vi "Host.vi"() -> ()   [LabVIEW 2018]
uses:
  <vilib>/userdefined/High Color/nirio_resource_hc.ctl
  <vilib>/FPGAPlugInAG/PXI-7953R/niLvFpga_Open_PXI-7953R.vi
  <vilib>/rvi/interface/common/dynamic/niFpgaDynamicAddResources.vi
  <vilib>/Utility/error.llb/Error Cluster From Error Code.vi
  <vilib>/rvi/errors/niLvFpgaAdjustHostInterfaceError.vi
  <vilib>/FPGAPlugInAG/Dynamic/niLvFpga_Close_Dynamic.vi
  <vilib>/rvi/interface/nirviOpenFPGA/nirviOpenFPGA.xnode
  FPGA Bitfiles/Memory_FPGATarget_Target_2uGpIeDGXOU.lvbitx
  <vilib>/rvi/interface/nirviReadWriteControl/nirviReadWriteControl.xnode
  <vilib>/rvi/interface/nirviMethod/nirviMethod.xnode
  <vilib>/rvi/interface/nirviCloseFPGA/nirviCloseFPGA.xnode
  <vilib>/FPGAPlugInAG/Dynamic/niLvFpga_ReadFifo_Dynamic.vi
  <vilib>/rvi/errors/niLvFpgaMergeErrorWithErrorCode.vi
  <vilib>/rvi/interface/Simulation/niFpgaSimulationCallBeginRW.vi
  NiFpgaLv.dll
panel:
  out "Data 2":u32[][](array[numeric])
  in  "Requested Number of Elements":u32
  in  "16384":u32
  in  "131":i32
  in  "Чтение всей памяти":bool
  out "Elements Remaining":u32
  out "Number of Elements to Write":u32
  out "Data":u8
  in  "2":u8=2
  in  "4":u8=4
  in  "Address":u32
  in  "Запись в DRAM":bool
  in  "D-0":u32
  in  "Чтение DRAM":bool
  in  "FIFO":bool
  in  "resource name":T1="PXI1Slot5" caption="RIO Device"
  in  "Стоп":bool
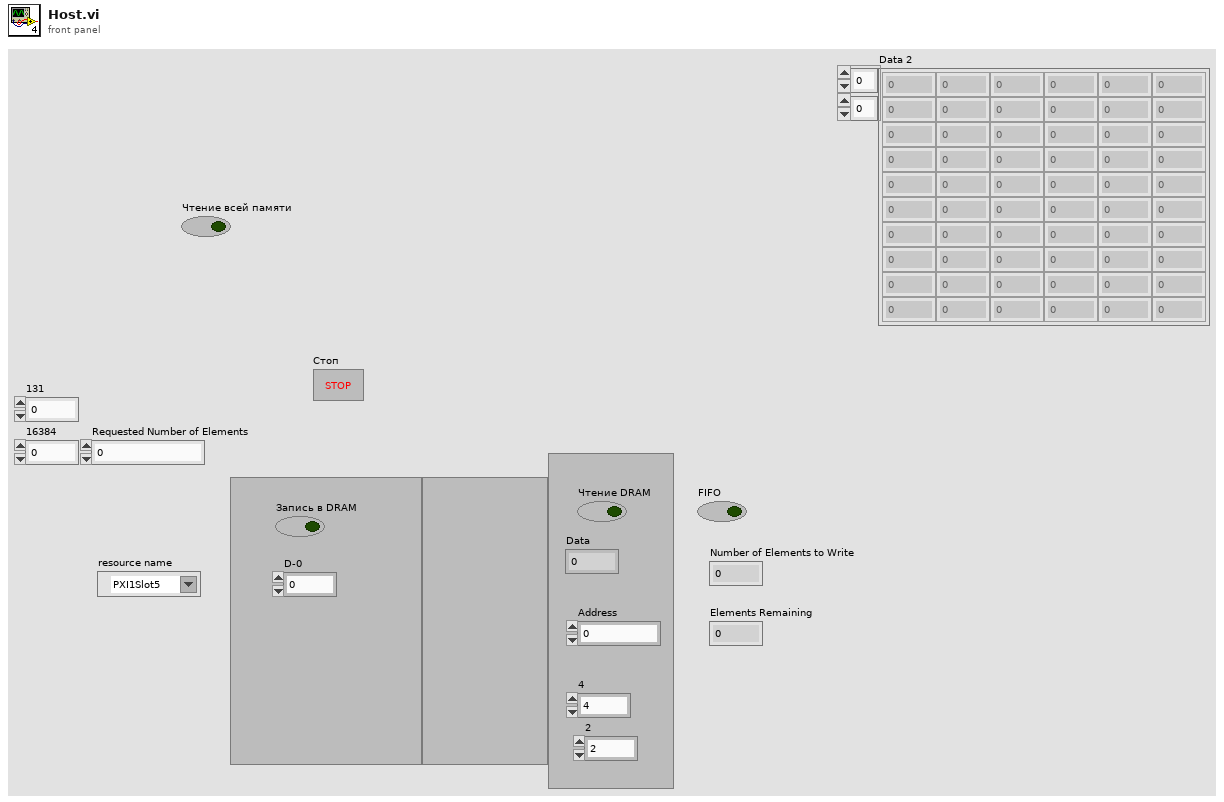
[diagram p1: front panel]
types:
  T1 = typedef "nirio_resource_hc.ctl" = tag
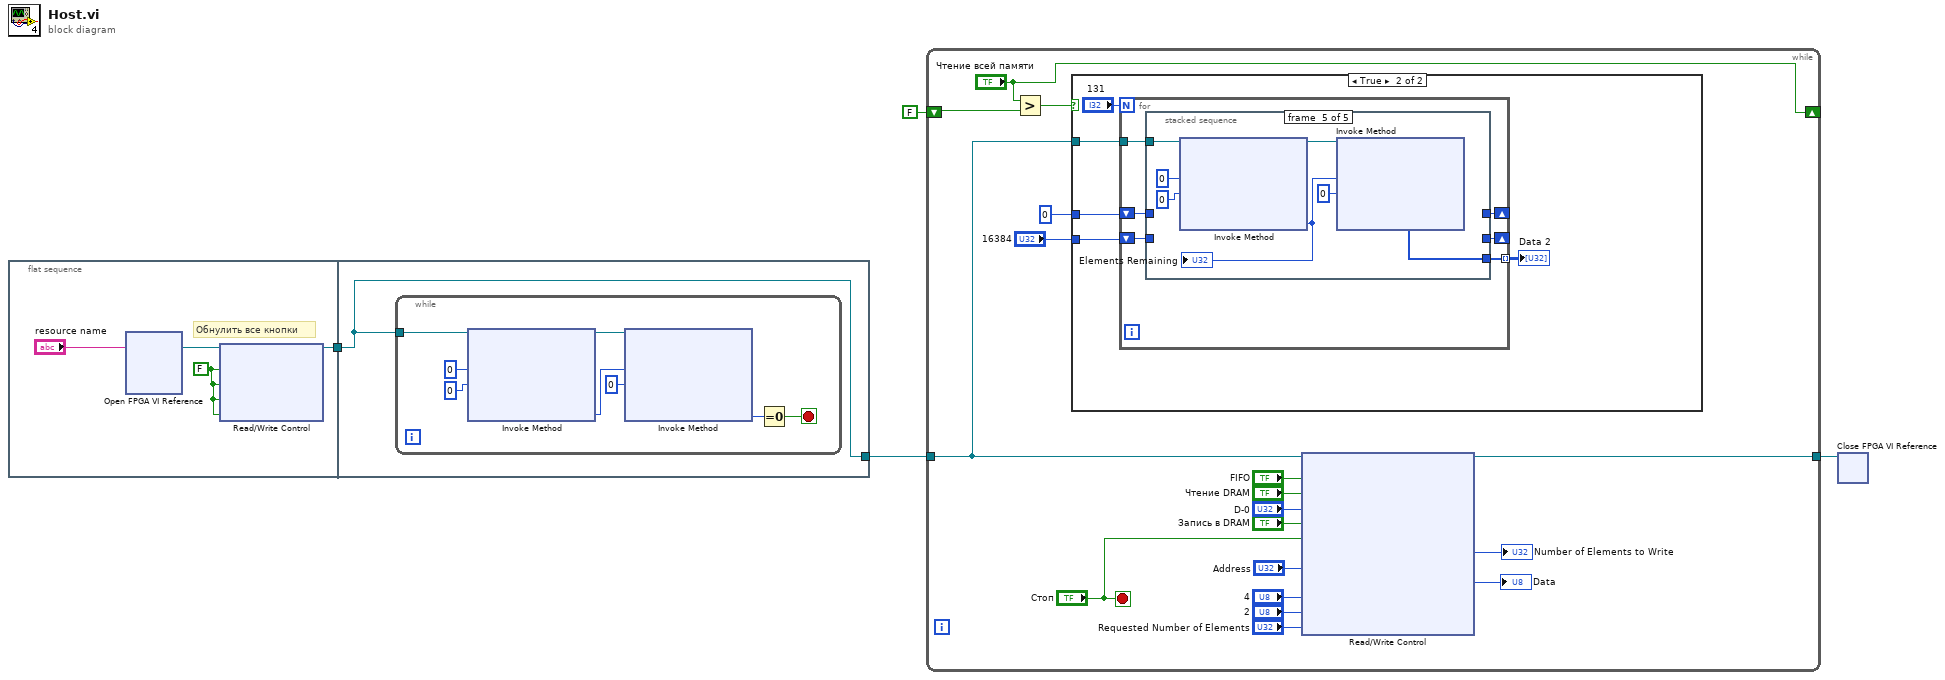
[diagram p0: block diagram]
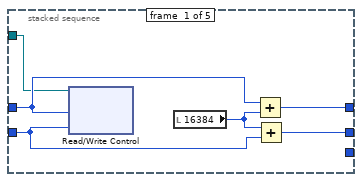
[diagram p3: hidden frame]
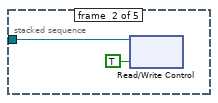
[diagram p4: hidden frame]
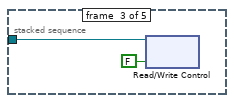
[diagram p5: hidden frame]
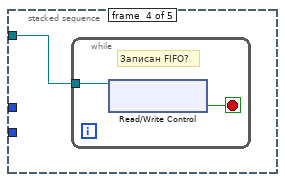
[diagram p6: hidden frame]
diagram:
  n1 = flat-sequence {
    tunnel: [w6] -> w1
    tunnel: [w9] -> w2
    tunnel: w1 -> [w9]
    frame #0 {
      w5 = FALSE
      # "Обнулить все кнопки"
      n2 = xnode "Open FPGA VI Reference"("resource name"="resource name") -> ("FPGA VI Reference Out"=w7:refnum<k20>)  [unwired: 1 in, 1 out]
      n3 = xnode "Read/Write Control"("FPGA VI Reference In"=w7, "FIFO"=w5, "Чтение DRAM"=w5, "HOST"=w5, "Запись в DRAM"=w5) -> ("FPGA VI Reference Out"=w6:refnum<k20>)  [unwired: 1 in, 1 out]
    }
    frame #1 {
      n4 = while {
        tunnel: w9 -> [w12]
        stop <- w11 stop-if-true
        n5 = xnode "Invoke Method"("FPGA VI Reference In"=w12, "Number of Elements"=u32 0, "Timeout (ms)"=0) -> ("FPGA VI Reference Out"=w14:refnum<k20>, "Elements Remaining"=w13:u32)  [unwired: 1 in, 2 out]
        n6 = xnode "Invoke Method"("FPGA VI Reference In"=w14, "Number of Elements"=w13, "Timeout (ms)"=0) -> ("Elements Remaining"=w10:u32)  [unwired: 1 in, 3 out]
        n7 = Equal To 0?(x=w10) -> (x = 0?=w11:bool)
      }
    }
  }
  n8 = while {
    tunnel: [w20] -> w4
    shift-right: ["Чтение всей памяти"] -> _
    shift-left: FALSE ("Чтение всей памяти") -> [w35]
    tunnel: w2 -> [w19]
    stop <- "Стоп" stop-if-true
    n9 = Greater?(x="Чтение всей памяти", y=w35) -> (0:w33:bool)
    n10 = case shown="True" w33 {
      tunnel: u32 0 -> [_ w39]
      tunnel: "16384" -> [_ w38]
      tunnel: w19 -> [_ w37]
      frame False {
      }
      frame True {
        n11 = for {
          N: "131" -> [_]
          tunnel: [w46] -> w36 mode=indexing
          shift-right: [w43] -> _
          shift-left: w39 -> [w45]
          shift-right: [w42] -> _
          shift-left: w38 -> [w44]
          tunnel: w37 -> [w41]
          n12 = stacked-sequence {
            tunnel: [_ _ _ _ w61] -> w46
            tunnel: w45 -> [w48 _ _ _ _]
            tunnel: w44 -> [w49 _ _ _ _]
            tunnel: [w51 _ _ _ _] -> w43
            tunnel: [w50 _ _ _ _] -> w42
            tunnel: w41 -> [w47 w54 w56 w57 w60]
            frame #0 {
              n13 = xnode "Read/Write Control"("FPGA VI Reference In"=w47, "Нач_адр"=w48, "Кон_адр"=w49) -> ()  [unwired: 1 in, 2 out]
              n14 = local read "16384"() -> (w52:u32)
              n15 = Add(x=w48, y=w52) -> (x+y=w51:u32)
              n16 = Add(x=w52, y=w49) -> (x+y=w50:u32)
            }
            frame #1 {
              n17 = xnode "Read/Write Control"("FPGA VI Reference In"=w54, "HOST"=TRUE) -> ()  [unwired: 1 in, 2 out]
            }
            frame #2 {
              n18 = xnode "Read/Write Control"("FPGA VI Reference In"=w56, "HOST"=FALSE) -> ()  [unwired: 1 in, 2 out]
            }
            frame #3 {
              n19 = while {
                tunnel: w57 -> [w59]
                stop <- w58 stop-if-true
                # "Записан FIFO?"
                n20 = xnode "Read/Write Control"("FPGA VI Reference In"=w59) -> ("Записали FIFO"=w58:bool)  [unwired: 1 in, 2 out]
              }
            }
            frame #4 {
              n21 = xnode "Invoke Method"("FPGA VI Reference In"=w60, "Number of Elements"=u32 0, "Timeout (ms)"=0) -> ("FPGA VI Reference Out"=w65:refnum<k20>, "Elements Remaining"=w66:u32)  [unwired: 1 in, 2 out]
              "Elements Remaining" <- w66
              n22 = xnode "Invoke Method"("FPGA VI Reference In"=w65, "Number of Elements"=w66, "Timeout (ms)"=0) -> ("Data"=w61:u32[])  [unwired: 1 in, 3 out]
            }
          }
        }
        "Data 2" <- w36
      }
    }
    n23 = xnode "Read/Write Control"("FPGA VI Reference In"=w19, "FIFO"="FIFO", "Чтение DRAM"="Чтение DRAM", "D-0"="D-0", "Запись в DRAM"="Запись в DRAM", "Стоп"="Стоп", "Address"="Address", "4"="4", "2"="2", "2097152"="Requested Number of Elements") -> ("FPGA VI Reference Out"=w20:refnum<k20>, "Number of Elements to Write"=→"Number of Elements to Write":u32, "Data"=→"Data":u8)  [unwired: 1 in, 1 out]
  }
  n24 = xnode "Close FPGA VI Reference"("FPGA VI Reference In"=w4) -> ()  [unwired: 1 in, 1 out]
